vi "Dequeue Message.vi"(0 "Message Queue In":refnum<queue>, 5 "Timeout":i32=60000, 11 "error in (no error)":errorcluster) -> (4 "Message Queue Out":refnum<queue>, 6 "Message Id":string, 8 "Message Data":variant, 10 "Timed Out":bool, 15 "error out":errorcluster)   [LabVIEW 2023, in "HAF.lvlib"]
doc: "Removes a message from the queue. If not message found in Timeout milliseconds then returns nothing. Default is to wait 60 seconds."
uses:
  HAF.lvlib
  Message.ctl
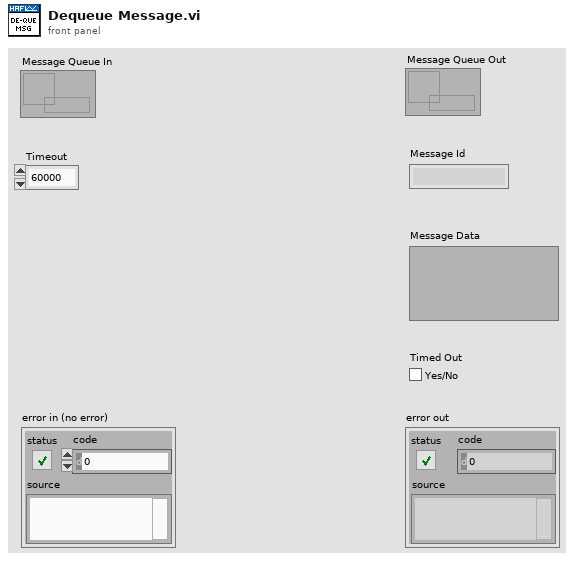
[diagram p1: front panel]
types:
  T1 = typedef "HAF.lvlib/Message.ctl" = cluster{"Message Id":string, "Message Data":variant}
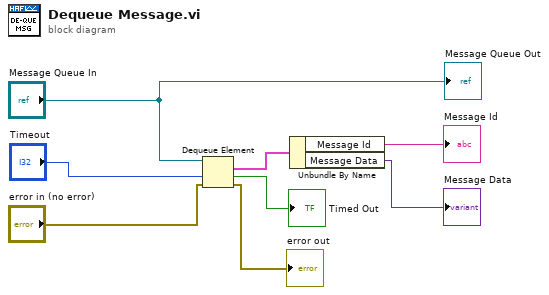
[diagram p0: block diagram]
diagram:
  n1 = Dequeue Element(queue="Message Queue In", timeout in ms (-1)="Timeout", error in (no error)="error in (no error)") -> (element=w6:T1, timed out?=→"Timed Out":bool, error out=→"error out":errorcluster)  [unwired: 1 out]
  n2 = Unbundle By Name(w6) -> ("Message Id"=→"Message Id":string, "Message Data"=→"Message Data":variant)
  "Message Queue Out" <- "Message Queue In"
